vi "GetLastErrorMessage.vi"(8 "error in (no error)":errorcluster, 11 "session id in":i32) -> (0 "error out":errorcluster, 1 "LastErrorMessage":string, 2 "isOk":bool, 3 "session id out":i32)   [LabVIEW 2017, in "libonnx_wrapper.lvlib"]
doc: "/**\n * @brief Получить последнее сообщение об ошибке для сессии\n * \n * Возвращает детальное текстовое описание последней ошибки, произошедшей\n * при работе с сессией (загрузка, инференс и т.д.).\n * \n * @param sessionId [IN] ID сессии\n * @param buffer [OUT] Буфер для строки с сообщением об ошибке\n * @param bufferSize [IN] Размер буфера (рекомендуется 512 или больше)\n * \n * @return int32: 0 при успехе\n * @return int32: -1 если сессия не найдена\n * \n * @note Если ошибок не было, вернет \"No error\"\n * @note Сообщение сохраняется до вызова ClearLastError или DestroySession\n */\nint GetLastErrorMessage(int sessionId, char* buffer, int bufferSize);"
uses:
  libonnx_wrapper.lvlib
panel:
  out "bufferSize":i32
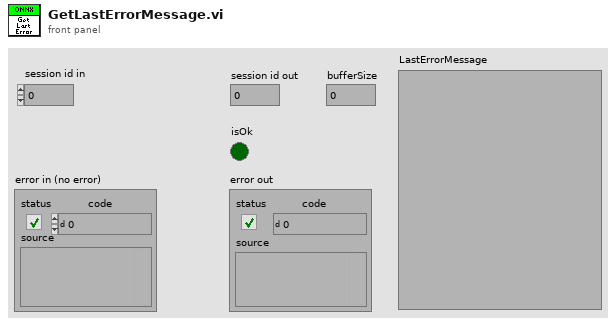
[diagram p1: front panel]
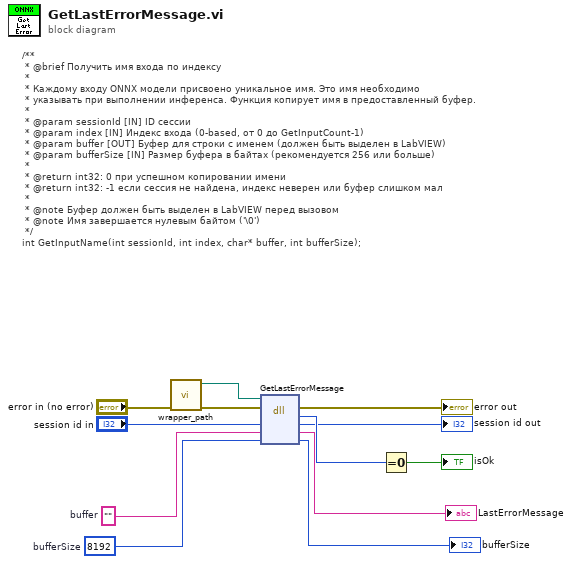
[diagram p0: block diagram]
diagram:
  w9 = 8192  # bufferSize
  w11 = ""  # buffer
  # "/**\n * @brief Получить имя входа по индексу\n * \n * Каждому входу ONNX модели присвоено уникальное имя. Это имя необходимо\n * указывать при выполнении инференса. Функция копирует имя в предоставленный буфер.\n * \n * @param sessionId [IN] ID сессии\n * @param index [IN] Индекс входа (0-based, от 0 до GetInputCount-1)\n * @param buffer [OUT] Буфер для строки с именем (должен быть выделен в LabVIEW)\n * @param bufferSize [IN] Размер буфера в байтах (рекомендуется 256 или больше)\n * \n * @return int32: 0 при успешном копировании имени\n * @return int32: -1 если сессия не найдена, индекс неверен или буфер слишком мал\n * \n * @note Буфер должен быть выделен в LabVIEW перед вызовом\n * @note Имя завершается нулевым байтом ('\\0')\n */\nint GetInputName(int sessionId, int index, char* buffer, int bufferSize);"
  n1 = call "wrapper_path.vi"("error in (no error)"="error in (no error)") -> ("error out"=w4:errorcluster, "wrapper path"=w7:path)  [unwired: 9 in]
  n2 = dll-call lib="home/ivan/LabVIEWData/ONNX/Test/libonnx_wrapper/unix64/libonnx_wrapper.so" fn="GetLastErrorMessage"(path in=w7, error in=w4, "sessionId"="session id in", "buffer"=w11, "bufferSize"=w9) -> (error out=→"error out":errorcluster, "GetLastErrorMessage"=w12:i32, "sessionId"=→"session id out":i32, "buffer"=→"LastErrorMessage":string, "bufferSize"=→"bufferSize":i32)  [unwired: 1 in, 1 out]
  n3 = Equal To 0?(x=w12) -> (x = 0?=→"isOk":bool)
